vi "SendCmd2.vi"(8 "error in (no error)":errorcluster, 11 "DataIn":string) -> (0 "error out":errorcluster, 2 "TimeOut":bool, 3 "Reccmd":string)   [LabVIEW 2015]
uses:
  Function/RobotCtrl Folder/Global/SN_Global.vi
panel:
  out "SN2":string
  out "SN1":string
  out "OffReply":string
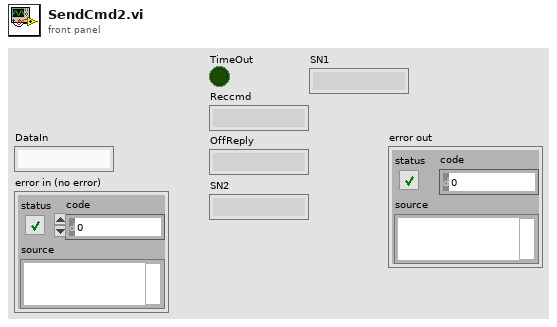
[diagram p1: front panel]
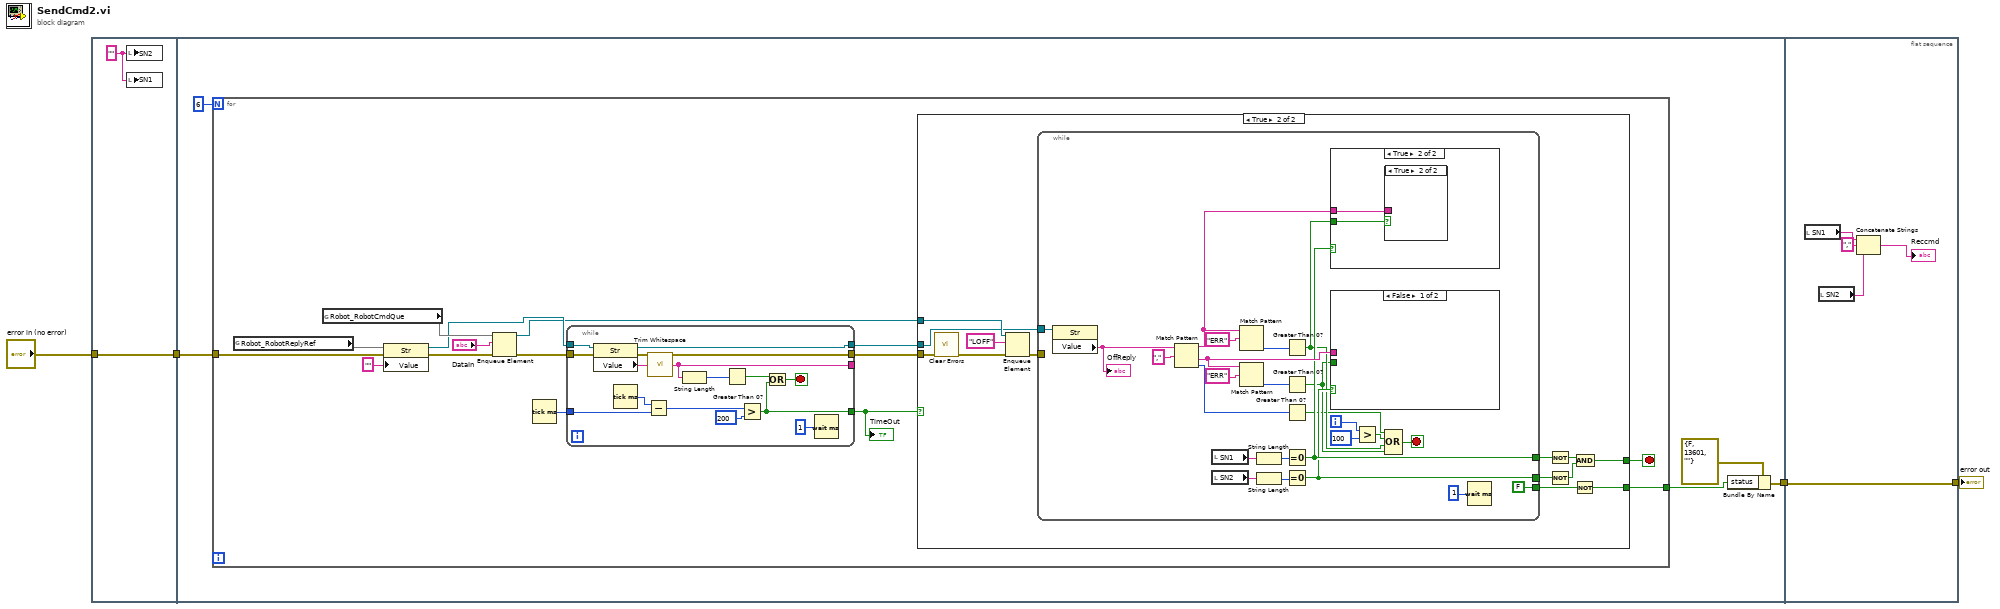
[diagram p0: block diagram]
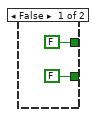
[diagram p2: hidden frame]
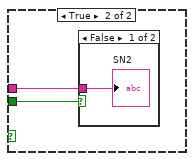
[diagram p3: hidden frame]
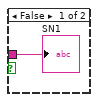
[diagram p6: hidden frame]
diagram:
  n1 = flat-sequence {
    tunnel: "error in (no error)" -> [w6]
    tunnel: [w6] -> w2
    tunnel: w2 -> [w11]
    tunnel: [w10] -> w1
    tunnel: [w92] -> w3
    tunnel: w1 -> [w92]
    frame #0 {
      w5 = "" ("SN2")
      n2 = local write "SN2"(w5) -> ()
      n3 = local write "SN1"(w5) -> ()
    }
    frame #1 {
      n4 = for {
        N: 6 -> [_]
        tunnel: w11 -> [w21]
        tunnel: [w13] -> w8
        stop <- w12 stop-if-true
        n5 = global read "SN_Global.vi" "Robot_RobotReplyRef"() -> (w24)
        n6 = global read "SN_Global.vi" "Robot_RobotCmdQue"() -> (w26)
        n7 = property class="Str"(reference=w24, error in=w21, "Value"="") -> (reference out=w20:refnum<vi>, error out=w22:errorcluster)
        n8 = Enqueue Element(queue=w26, element="DataIn", error in (no error)=w22) -> (queue out=w17:refnum<queue>, error out=w18:errorcluster)  [unwired: 1 in, 1 out]
        n9 = Tick Count (ms)() -> (millisecond timer value=w19:u32)
        n10 = while {
          tunnel: w20 -> [w86]
          tunnel: w19 -> [w84]
          tunnel: w18 -> [w78]
          tunnel: [w77] -> w16
          tunnel: [w76] -> w14
          tunnel: [w75] -> _
          tunnel: [w73] -> w15
          stop <- w79 stop-if-true
          n11 = property class="Str"(reference=w86, error in=w78) -> (reference out=w73:refnum<vi>, error out=w77:errorcluster, "Value"=w87:string)
          n12 = Tick Count (ms)() -> (millisecond timer value=w83:u32)
          n13 = Subtract(x=w83, y=w84) -> (x-y=w82:u32)
          n14 = call <vilib>:"Trim Whitespace.vi"("string"=w87) -> ("trimmed string"=w75:string)  [unwired: 1 in]
          n15 = String Length(string=w75) -> (length=w85:i32)
          n16 = Greater Than 0?(x=w85) -> (x > 0?=w80:bool)
          n17 = Greater?(x=w82, y=u32 200) -> (0:w76:bool)
          n18 = Or(x=w80, y=w76) -> (x .or. y?=w79:bool)
          n19 = Wait (ms)(milliseconds to wait=u32 1 ("millisecond timer value")) -> ()  [unwired: 1 out]
        }
        "TimeOut" <- w14
        n20 = case shown="True" w14 {
          tunnel: w17 -> [_ w41]
          tunnel: w16 -> [_ w39]
          tunnel: w15 -> [_ w37]
          tunnel: [FALSE w34] -> w13
          tunnel: [FALSE w29] -> w12
          frame False {
          }
          frame True {
            n21 = call <vilib>:"Clear Errors.vi"("error in (no error)"=w39) -> ("error out"=w38:errorcluster)  [unwired: 5 in, 1 out]
            n22 = Enqueue Element(queue=w41, element="LOFF", error in (no error)=w38) -> (error out=w36:errorcluster)  [unwired: 1 in, 2 out]
            n23 = while {
              tunnel: w37 -> [w66]
              tunnel: w36 -> [_]
              tunnel: [FALSE] -> w35
              tunnel: [w49] -> w33
              tunnel: [w48] -> w32
              i -> [w64]
              stop <- w46 stop-if-true
              n24 = property class="Str"(reference=w66) -> ("Value"=w61:string)  [unwired: 1 in, 2 out]
              "OffReply" <- w61
              n25 = Match Pattern(string=w61, regular expression=",") -> (before substring=w54:string, after substring=w55:string, offset past match=w43:i32)  [unwired: 1 in, 1 out]
              n26 = local read "SN1"() -> (w53:string)
              n27 = local read "SN2"() -> (w50:string)
              n28 = Match Pattern(string=w54, regular expression="ERR") -> (offset past match=w57:i32)  [unwired: 1 in, 3 out]
              n29 = Match Pattern(string=w55, regular expression="ERR") -> (offset past match=w56:i32)  [unwired: 1 in, 3 out]
              n30 = String Length(string=w53) -> (length=w52:i32)
              n31 = String Length(string=w50) -> (length=w51:i32)
              n32 = Greater Than 0?(x=w57) -> (x > 0?=w45:bool)
              n33 = Greater Than 0?(x=w56) -> (x > 0?=w44:bool)
              n34 = Greater Than 0?(x=w43) -> (x > 0?=w42:bool)
              n35 = Equal To 0?(x=w52) -> (x = 0?=w49:bool)
              n36 = Equal To 0?(x=w51) -> (x = 0?=w48:bool)
              n37 = case shown="True" w49 {
                tunnel: w45 -> [_ w71]
                tunnel: w54 -> [_ w70]
                frame False {
                }
                frame True {
                  n38 = case shown="True" w71 {
                    tunnel: w70 -> [w72 _]
                    frame False {
                      "SN1" <- w72
                    }
                    frame True {
                    }
                  }
                }
              }
              n39 = case shown="False" w48 {
                tunnel: w44 -> [_ w68]
                tunnel: w55 -> [_ w67]
                frame False {
                }
                frame True {
                  n40 = case shown="False" w68 {
                    tunnel: w67 -> [w69 _]
                    frame False {
                      "SN2" <- w69
                    }
                    frame True {
                    }
                  }
                }
              }
              n41 = Greater?(x=w64, y=100) -> (0:w62:bool)
              n42 = Compound Arithmetic op=OR(w42, w62, w45, w44) -> (w46:bool)
              n43 = Wait (ms)(milliseconds to wait=u32 1 ("millisecond timer value")) -> ()  [unwired: 1 out]
            }
            n44 = Not(x=w33) -> (.not. x?=w31:bool)
            n45 = Not(x=w32) -> (.not. x?=w30:bool)
            n46 = Not(x=w35) -> (.not. x?=w34:bool)
            n47 = And(x=w31, y=w30) -> (x .and. y?=w29:bool)
          }
        }
      }
      n48 = Bundle By Name(cluster=errorcluster {"status"=FALSE, "code"=13601, "source"=""} ("error constant"), "status"=w8) -> (w10:errorcluster)
    }
    frame #2 {
      n49 = local read "SN1"() -> (w91:string)
      n50 = local read "SN2"() -> (w89:string)
      n51 = Concatenate Strings(w91, "," ("string"), w89) -> (→"Reccmd":string)
    }
  }
  "error out" <- w3
